vi "Read HSMS Class.vi"(8 "error in (no error)":errorcluster, 11 "Scenarios Class in":refnum<class "Scenarios Class.lvclass">) -> (0 "error out":errorcluster, 2 "HSMS Class":refnum<class "HSMS Class.lvclass">, 3 "Scenarios Class out":refnum<class "Scenarios Class.lvclass">)   [LabVIEW 2020, in "SECS Scenarios.lvlib" / "Scenarios Class.lvclass"]
uses:
  Scenarios Class.lvclass
  SECS Communication/HSMS Class/HSMS Class.lvclass
  Scenarios Class.lvclass/Scenarios Class.ctl
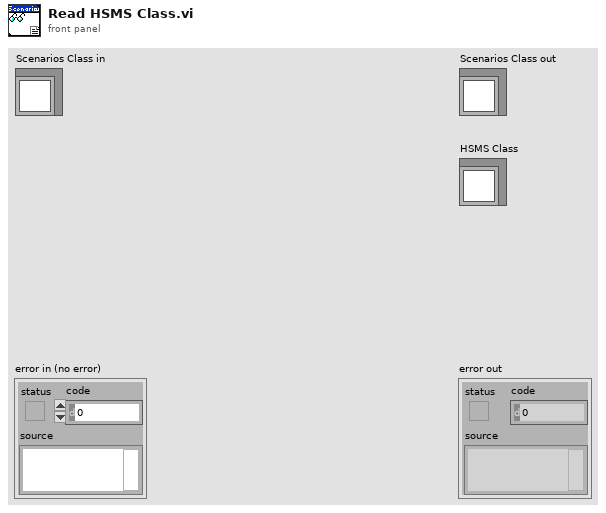
[diagram p1: front panel]
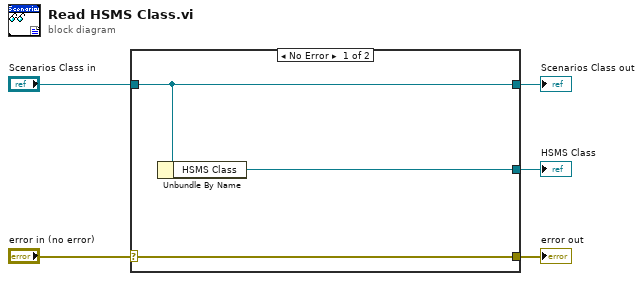
[diagram p0: block diagram]
diagram:
  n1 = case shown="No Error" "error in (no error)" {
    selector: "error in (no error)" -> [w8 w9]
    tunnel: [w8 w9] -> w4
    tunnel: [w7 w10] -> w2
    tunnel: "Scenarios Class in" -> [w7 w10]
    tunnel: [w6 _] -> w1
    frame No Error {
      n2 = Unbundle By Name(w7) -> ("HSMS Class"=w6:refnum<class "HSMS Class.lvclass">)
    }
    frame Error {
    }
  }
  "error out" <- w4
  "Scenarios Class out" <- w2
  "HSMS Class" <- w1
